vi "MainGui.Buttons.GetState.vi"(0 "Button":T1=enum."Stop", 1 "Btns":refnum<vi>[](array[refnum])) -> (2 "State":bool)   [LabVIEW 2016]
uses:
  MainGui.ButtonType.ctl
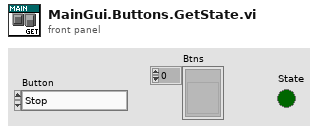
[diagram p1: front panel]
types:
  T1 = typedef "MainGui.ButtonType.ctl" = enum32{"Exit", "Mode", "Process", "Base", "Order", "Manual", "Logs", "Results", "Accept", "Reject", "Start", "Stop", "Next", "Pause", "Lock", "ManualView", "DoorLock", "Scan", "Select", "ScannerGui", "Stats"}
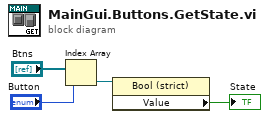
[diagram p0: block diagram]
diagram:
  n1 = Index Array(array="Btns", index="Button") -> (element=w2:refnum<vi>)
  n2 = property class="Bool (strict)"(reference=w2) -> ("Value"=→"State":bool)  [unwired: 1 in, 2 out]
